vi "ExponentialSmoothing.vi"(10 "Smoothing Factor":dbl, 11 "Value":dbl) -> (3 "Smooth Value":dbl)   [LabVIEW 2018]
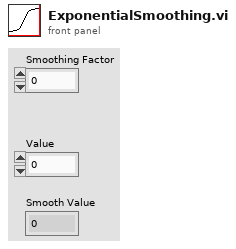
[diagram p1: front panel]
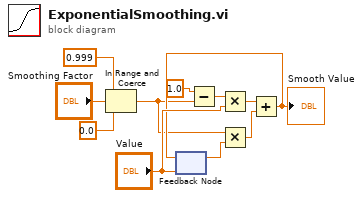
[diagram p0: block diagram]
diagram:
  n1 = In Range and Coerce(upper limit=0.999, x="Smoothing Factor", lower limit=0.0) -> (coerced(x)=w3:dbl)  [unwired: 1 out]
  n2 = feedback #1("Value") -> (w6:dbl)
  n3 = Subtract(x=1.0, y=w3) -> (x-y=w10:dbl)
  n4 = Multiply(x=w10, y="Value") -> (x*y=w9:dbl)
  n5 = Multiply(x=w3, y=w6) -> (x*y=w5:dbl)
  n6 = Add(x=w9, y=w5) -> (x+y=w4:dbl)
  "Smooth Value" <- w4
  n7 = feedback-in #1(w4) -> ()
